vi "Emballage_fichierSpecifique_S0020002_HTML.vi"(5 "Indice Rev. Client":string, 6 "Logo IMI (U:\\MTD_PRD_TESTS\\PARAM_TESTS\\EMBALLAGE\\LogoIMI.JPG)":path=path "U:/MTD_PRD_TESTS/PARAM_TESTS/EMBALLAGE/LogoIMI.JPG", 7 "N° article client":string, 8 "Error in":errorcluster caption="Error in (no error)", 9 "PDF filename path":path=path "C:/Users/ltinguely/Desktop/test.pdf", 10 "report file path":path=path "C:/Users/ltinguely/Desktop/test.html" caption="chemin du fichier du rapport", 11 "Tableau n° valves":string[](array[string])=["100200021121130326", "100200021121130308", "100200021121130314", "100200021121130316", "100200021121130319", "100200021121130330", "100200021121130309", "100200021121130307", "100200021121130311", "100200021121130299", "100200021121130310", "100200021121130313", "100200021121130321", "100200021121130336", "100200021121130322", "100200021121130302", "100200021121130334", "100200021121130317", "100200021121130348", "100200021121130333", "100200021121130355", "100200021121130345", "100200021121130349", "100200021121130350", "100200021121130315", "100200021121130352", "100200021121130328", "100200021121130337", "100200021121130357", "100200021121130359", "100200021121130360", "100200021121130344", "100200021121130347", "100200021121130358", "100200021121130341", "100200021121130338", "100200021121130331", "100200021121130329", "100200021121130332", "100200021121130339", "100200021121130340", "100200021121130343", "100200021121130351", "100200021121130354", "100200021121130346", "100200021121130335", "100200021121130342", "100200021121130353", "100200021121130383", "100200021121130384", "100200021121130380", "100200021121130389", "100200021121130382", "100200021121130379", "100200021121130376", "100200021121130378", "100200021121130391", "100200021121130392", "100200021121130372", "100200021121130362", "100200021121130375", "100200021121130371", "100200021121130385", "100200021121130364", "100200021121130386", "100200021121130361", "100200021121130366", "100200021121130365", "100200021121130367", "100200021121130363", "100200021121130377", "100200021121130374", "100200021121130369", "100200021121130370", "100200021121130373", "100200021121130388", "100200021121130368", "100200021121130356", "100200021121130412", "100200021121130407", "100200021121130406", "100200021121130408", "100200021121130398", "100200021121130415", "100200021121130402", "100200021121130399", "100200021121130414", "100200021121130413", "100200021121130393", "100200021121130390", "100200021121130403", "100200021121130401", "100200021121130387", "100200021121130381", "100200021121130395", "100200021121130394", "100200021121130411", "100200021121130410", "100200021121130405", "100200021121130396", "100200021121130397", "100200021121130400", "100200021121130404", "100200021121130211", "100200021121130215", "100200021121130217", "100200021121130212", "100200021121130219", "100200021121130225", "100200021121130213", "100200021121130216", "100200021121130226", "100200021121130224", "100200021121130223", "100200021121130230", "100200021121130220", "100200021121130214", "100200021121130229", "100200021121130236", "100200021121130238", "100200021121130239", "100200021121130237", "100200021121130234", "100200021121130242", "100200021121130241", "100200021121130233", "100200021121130210", "100200021121130218", "100200021121130240", "100200021121130221", "100200021121130245", "100200021121130222", "100200021121130235", "100200021121130247", "100200021121130227", "100200021121130231", "100200021121130228", "100200021121130243", "100200021121130246", "100200021121130251", "100200021121130273", "100200021121130267", "100200021121130268", "100200021121130256", "100200021121130265", "100200021121130261", "100200021121130264", "100200021121130254", "100200021121130257", "100200021121130249", "100200021121130248", "100200021121130250", "100200021121130244", "100200021121130253", "100200021121130266", "100200021121130252", "100200021121130274", "100200021121130263", "100200021121130232", "100200021121130262", "100200021121130260", "100200021121130269", "100200021121130270", "100200021121130294", "100200021121130255", "100200021121130258", "100200021121130295", "100200021121130297", "100200021121130291", "100200021121130289", "100200021121130278", "100200021121130283", "100200021121130284", "100200021121130296", "100200021121130277", "100200021121130286", "100200021121130288", "100200021121130287", "100200021121130275", "100200021121130290", "100200021121130298", "100200021121130279", "100200021121130292", "100200021121130259", "100200021121130293", "100200021121130272", "100200021121130271", "100200021121130276", "100200021121130282", "100200021121130281", "100200021121130280", "100200021121130285", "100200021121130300", "100200021121130152", "100200021121130165", "100200021121130178", "100200021121130151", "100200021121130175", "100200021121130173", "100200021121130157", "100200021121130167", "100200021121130155", "100200021121130174", "100200021121130164", "100200021121130163", "100200021121130159", "100200021121130160", "100200021121130186", "100200021121130154", "100200021121130169", "100200021121130166", "100200021121130156", "100200021121130207", "100200021121130192", "100200021121130158", "100200021121130161", "100200021121130168", "100200021121130170", "100200021121130171", "100200021121130162", "100200021121130190", "100200021121130191", "100200021121130193", "100200021121130182", "100200021121130183", "100200021121130176", "100200021121130148", "100200021121130177", "100200021121130203", "100200021121130184", "100200021121130189", "100200021121130194", "100200021121130179", "100200021121130196", "100200021121130188", "100200021121130180", "100200021121130187", "100200021121130181", "100200021121130195", "100200021121130185", "100200021121130204", "100200021121130202", "100200021121130200", "100200021121130198", "100200021121130197", "100200021121130199", "100200021121130150", "100200021121130111", "100200021121130201", "100200021121130208", "100200021121130209", "100200021121130205", "100200021121130206", "100200021121130093", "100200021121130091", "100200021121130109", "100200021121130088", "100200021121130099", "100200021121130097", "100200021121130096", "100200021121130102", "100200021121130095", "100200021121130092", "100200021121130094", "100200021121130098", "100200021121130101", "100200021121130100", "100200021121130106", "100200021121130121", "100200021121130104", "100200021121130107", "100200021121130089", "100200021121130103", "100200021121130105", "100200021121130108", "100200021121130120", "100200021121130125", "100200021121130138", "100200021121130114", "100200021121130115", "100200021121130119", "100200021121130118", "100200021121130117", "100200021121130113", "100200021121130112", "100200021121130124", "100200021121130110", "100200021121130116", "100200021121130149", "100200021121130145", "100200021121130127", "100200021121130130", "100200021121130128", "100200021121130129", "100200021121130134", "100200021121130133", "100200021121130135", "100200021121130143", "100200021121130139", "100200021121130147", "100200021121130136", "100200021121130141", "100200021121130144", "100200021121130126", "100200021121130123", "100200021121130122", "100200021121130132", "100200021121130131", "100200021121130140", "100200021121130146", "100200021121130137", "100200021121130142", "100200021121130153", "100200021121130060", "100200021121130077", "100200021121130059", "100200021121130040", "100200021121130075", "100200021121130082", "100200021121130022", "100200021121130086", "100200021121130045", "100200021121130078", "100200021121130080", "100200021121130074", "100200021121130065", "100200021121130066", "100200021121130070", "100200021121130068", "100200021121130084", "100200021121130069", "100200021121130076", "100200021121130081", "100200021121130083", "100200021121130085", "100200021121130087", "100200021121130090", "100200021121130012", "100200021121130028", "100200021121130079", "100200021121130073", "100200021121130072", "100200021121130071", "100200021121130042", "100200021121130030", "100200021121130033", "100200021121130032", "100200021121130027", "100200021121130031", "100200021121130025", "100200021121130020", "100200021121130026", "100200021121130003", "100200021121130008", "100200021121130001", "100200021121130019", "100200021121120509", "100200021121130021", "100200021121130016", "100200021121130013", "100200021121120510", "100200021121130015", "100200021121130002", "100200021121130014", "100200021121130029", "100200021121130049", "100200021121130048", "100200021121130011", "100200021121130063", "100200021121130009", "100200021121130010", "100200021121130004", "100200021121130017", "100200021121130018", "100200021121130024", "100200021121130023", "100200021121130061", "100200021121130062", "100200021121130064", "100200021121130058", "100200021121130046", "100200021121130056", "100200021121130057", "100200021121130054", "100200021121130051", "100200021121130044", "100200021121130035", "100200021121130043", "100200021121130005", "100200021121130038", "100200021121130039", "100200021121130047", "100200021121130053", "100200021121130007", "100200021121130037", "100200021121130006", "100200021121130052", "100200021121130041", "100200021121130034", "100200021121130036", "100200021121130067", "100200021121130050", "100200021121130055", "100200021121120410", "100200021121120406", "100200021121120421", "100200021121120408", "100200021121120424", "100200021121120416", "100200021121120423", "100200021121120419", "100200021121120407", "100200021121120397", "100200021121120396", "100200021121120404", "100200021121120422", "100200021121120392", "100200021121120403", "100200021121120405", "100200021121120400", "100200021121120385", "100200021121120348", "100200021121120388", "100200021121120414", "100200021121120412", "100200021121120320", "100200021121120394", "100200021121120447", "100200021121120398", "100200021121120444", "100200021121120417", "100200021121120395", "100200021121120402", "100200021121120401", "100200021121120393", "100200021121120399", "100200021121120425", "100200021121120449", "100200021121120415", "100200021121120446", "100200021121120439", "100200021121120426", "100200021121120434", "100200021121120453", "100200021121120455", "100200021121120441", "100200021121120443", "100200021121120435", "100200021121120409", "100200021121120420", "100200021121120427", "100200021121120429", "100200021121120438", "100200021121120432", "100200021121120437", "100200021121120430", "100200021121120440", "100200021121120442", "100200021121120428", "100200021121120464", "100200021121120433", "100200021121120418", "100200021121120445", "100200021121120431", "100200021121120463", "100200021121120451", "100200021121120466", "100200021121120454", "100200021121120452", "100200021121120459", "100200021121120411", "100200021121120458", "100200021121120472", "100200021121120470", "100200021121120474", "100200021121120462", "100200021121120477", "100200021121120436", "100200021121120469", "100200021121120467", "100200021121120413", "100200021121120460", "100200021121120486", "100200021121120476", "100200021121120473", "100200021121120468", "100200021121120478", "100200021121120482", "100200021121120471", "100200021121120479", "100200021121120456", "100200021121120465", "100200021121120461", "100200021121120488", "100200021121120457", "100200021121120475", "100200021121120489", "100200021121120493", "100200021121120487", "100200021121120485"]) -> (0 "Error out":errorcluster, 1 "report out":refnum<class "NI_report.lvclass"> caption="rapport en sortie", 2 "path out":path, 3 "IsSuccessful":bool)   [LabVIEW 2020]
uses:
  <vilib>/Utility/NIReport.llb/NI_report.lvclass
  <vilib>/Utility/NIReport.llb/Report Type.ctl
  <vilib>/printing/OpenHTMLReport.llb/Open HTML Report in Browser (Refnum).vi
  <vilib>/Utility/NIReport.llb/NI_ReportGenerationCore.lvlib
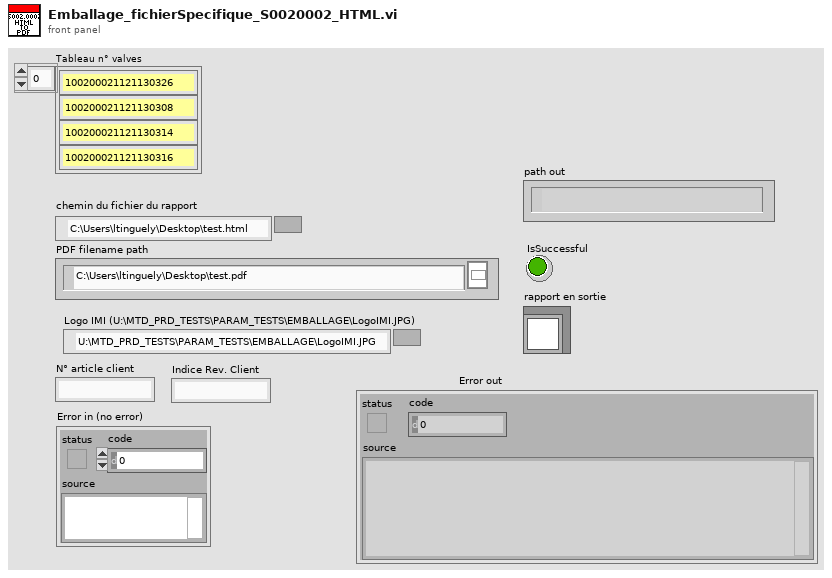
[diagram p1: front panel]
types:
  T1 = typedef "NI_ReportGenerationCore.lvlib/Report Type.ctl" = enum16{"HTML", "Word", "Excel"}
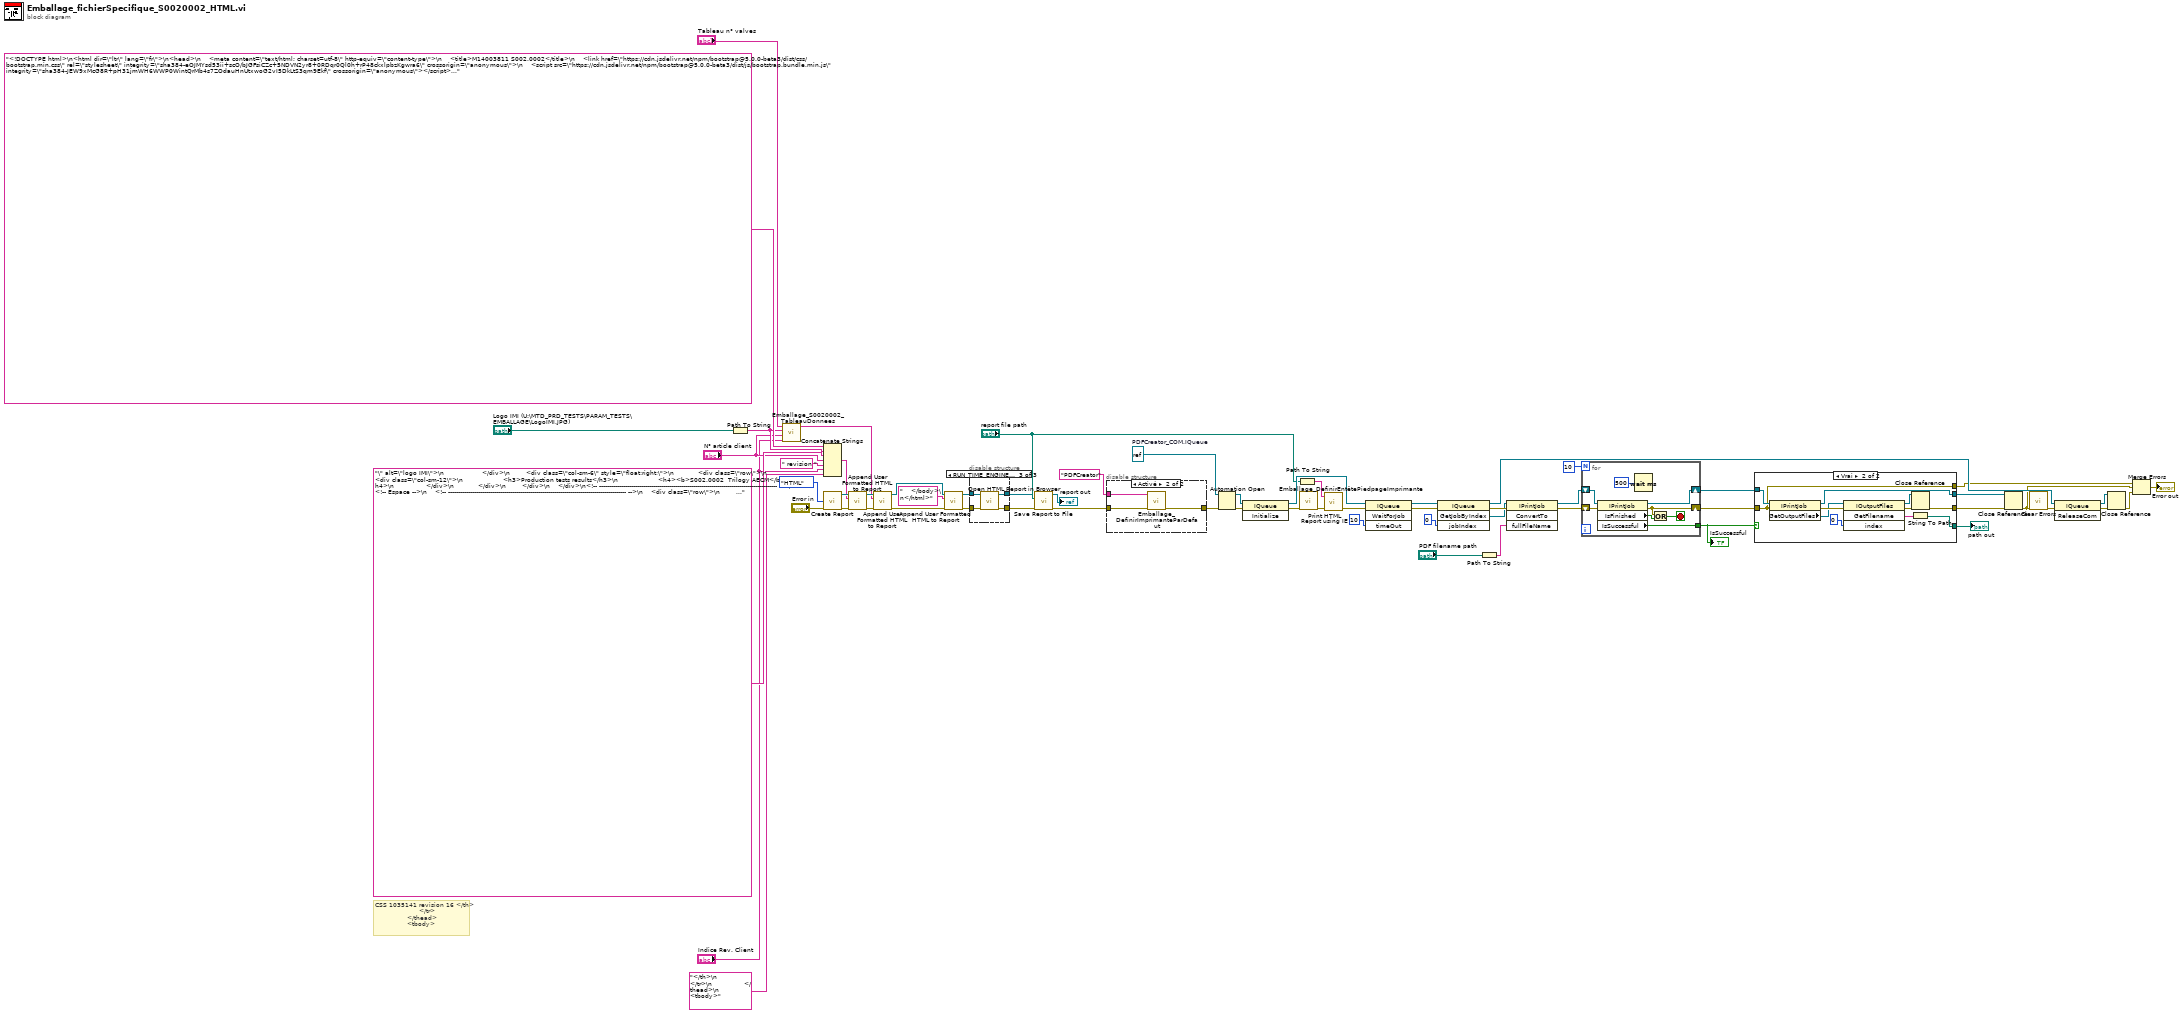
[diagram p0: block diagram]
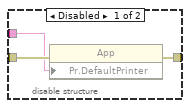
[diagram p2: hidden frame]
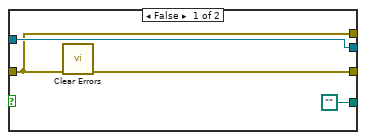
[diagram p5: hidden frame]
diagram:
  w52 = refnum<k7> refnum  # PDFCreator_COM.IQueue
  # "CSS 1035141 revision 16 </th>\n                      </tr>\n                </thead>\n                <tbody>"
  n1 = Path To String(path="Logo IMI (U:\\MTD_PRD_TESTS\\PARAM_TESTS\\EMBALLAGE\\LogoIMI.JPG)") -> (string=w20:string)
  n2 = call "Emballage_S0020002_TableauDonnees.vi"("Indice Rev Client"="Indice Rev. Client", "N° article client"="N° article client", "Chemin Logo"=w20, "Tableau n° valves"="Tableau n° valves") -> ("Chaîne en sortie"=w28:string)  [unwired: 7 in]
  n3 = Concatenate Strings("<!DOCTYPE html>\n<html dir=\"ltr\" lang=\"fr\">\n<head>\n    <meta content=\"text/html; charset=utf-8\" http-equiv=\"content-type\">\n    <title>M14003811 S002.0002</title>\n    <link href=\"https://cdn.jsdelivr.net/npm/bootstrap@5.0.0-beta3/dist/css/bootstrap.min.css\" rel=\"stylesheet\" integrity=\"sha384-eOJMYsd53ii+scO/bJGFsiCZc+5NDVN2yr8+0RDqr0Ql0h+rP48ckxlpbzKgwra6\" crossorigin=\"anonymous\">\n    <script src=\"https://cdn.jsdelivr.net/npm/bootstrap@5.0.0-beta3/dist/js/bootstrap.bundle.min.js\" integrity=\"sha384-JEW9xMcG8R+pH31jmWH6WWP0WintQrMb4s7ZOdauHnUtxwoG2vI5DkLtS3qm9Ekf\" crossorigin=\"anonymous\"></script>\n<style>\n        @media all {\n    table {\n        margin: auto;\n    }\n    table,\n    th,\n    td {\n        padding: 1px;\n        border: 1px solid black;\n        border-collapse: collapse;\ntext-align: center;\n    }\n}\n@media print {\ntable{\ndisplay:table !important;\n    width:80%;\n    margin-left:10%;\n}\n}\n      </style>\n       <meta content=\"LTinguely\" name=\"author\">\n    <meta content=\"M14003811\" name=\"description\">\n    <meta content=\"M14003811\" name=\"keywords\">\n</head>\n<body>\n    <!-- ----------------------------------------------------------------------------------------- -->\n    <!-- Titre -->\n    <!-- ----------------------------------------------------------------------------------------- -->\n     <div class=\"row\" style=\"display: inline-block\">\n        <div class=\"col-sm-6\" style=\"float:left;\">\n                            <img src=\"", w20, "\" alt=\"logo IMI\">\n                   </div>\n        <div class=\"col-sm-6\" style=\"float:right;\">\n            <div class=\"row\">\n                <div class=\"col-sm-12\">\n                    <h3>Production tests results</h3>\n                    <h4><b>S002.0002  Trilogy AECM</b></h4>\n                </div>\n            </div>\n        </div>\n    </div>\n<!-- ----------------------------------------------------------------------------------------- -->\n    <!-- Espace -->\n    <!-- ----------------------------------------------------------------------------------------- -->\n    <div class=\"row\">\n        <div class=\"col-sm-12\">\n            <br>\n            <br>\n        </div>\n    </div>\n    <!-- ----------------------------------------------------------------------------------------- -->\n    <!-- Explciation Fichier Encadrée -->\n    <!-- ----------------------------------------------------------------------------------------- -->\n    <div class=\"row border border-dark\">\n        <div class=\"col-sm-12\">\n            <p style=\"font-weight: bold;\">This document is a complementory document to the Certificate of Conformity.<br>\n            This document states the test result status (Pass or Fail) for each parts serial number for which\n            the associated certificate of Conformity was issued</p>\n        </div>\n    </div>\n    <!-- ----------------------------------------------------------------------------------------- -->\n    <!-- Espace -->\n    <!-- ----------------------------------------------------------------------------------------- -->\n    <div class=\"row\">\n        <div class=\"col-sm-12\">\n            <br>\n            <br>\n        </div>\n    </div>\n    <!-- ----------------------------------------------------------------------------------------- -->\n    <!-- Données -->\n    <!-- ----------------------------------------------------------------------------------------- -->\n    \n            <table>\n                <thead>\n                    <tr>\n                        <th></th>\n                        <th>Serial Number</th>\n                        <th>Test results according to<br>" ("HTML text"), "N° article client", " revision " ("chaîne"), "Indice Rev. Client", "</th>\n                      </tr>\n                </thead>\n                <tbody>" ("chaîne")) -> (w24:string)
  n4 = call <vilib>:"Create Report.vi"("report type"=Report_Type."HTML", "error in (no error)"="Error in") -> ("report out"=w25:refnum<class "NI_report.lvclass">, "error out"=w26:errorcluster)  [unwired: 12 in]
  n5 = call-dynamic "Append User Formatted HTML to Report.vi"("report in"=w25, "HTML text"=w24, "error in (no error)"=w26) -> ("report out"=w59:refnum<class "NI_report.lvclass">, "error out"=w60:errorcluster)  [unwired: 11 in]
  n6 = call-dynamic "Append User Formatted HTML to Report.vi"("report in"=w59, "HTML text"=w28, "error in (no error)"=w60) -> ("report out"=w58:refnum<class "NI_report.lvclass">, "error out"=w57:errorcluster)  [unwired: 11 in]
  n7 = call-dynamic "Append User Formatted HTML to Report.vi"("report in"=w58, "HTML text"="    </body>\n</html>", "error in (no error)"=w57) -> ("report out"=w19:refnum<class "NI_report.lvclass">, "error out"=w18:errorcluster)  [unwired: 11 in]
  n8 = disable-structure shown="RUN_TIME_ENGINE==False" {
    disable-tunnel: w19 -> [w64 w66 w70]
    disable-tunnel: w18 -> [w63 w65 w69]
    disable-tunnel: [w64 w66 w68] -> w17
    disable-tunnel: [w63 w65 w67] -> w16
    frame condition #0 {
    }
    frame condition #1 {
    }
    frame condition #2 (active) {
      n9 = call-poly <vilib>:"Open HTML Report in Browser.vi"("report in"=w70, "error in (no error)"=w69) -> ("report out"=w68:refnum<class "NI_report.lvclass">, "error out"=w67:errorcluster)  [unwired: 11 in, 1 out]
    }
  }
  n10 = call-dynamic "Save Report to File.vi"("report in"=w17, "report file path"="report file path", "error in (no error)"=w16) -> ("report out"=→"report out":refnum<class "NI_report.lvclass">, "error out"=w6:errorcluster)  [unwired: 11 in]
  n11 = disable-structure shown="Activé" {
    disable-tunnel: [w73 w74] -> w53
    disable-tunnel: w6 -> [w72 w75]
    disable-tunnel: "PDFCreator" ("Printing:Default Printer") -> [w71 w76]
    frame Disabled {
      n12 = property class="App"(error in=w72, "Pr.DefaultPrinter"=w71) -> (error out=w73:errorcluster)  [unwired: 1 in, 1 out]
    }
    frame Enabled {
      n13 = call "Emballage_DefinirImprimanteParDefaut.vi"("Error in"=w75, "Imprimante"=w76) -> ("Error out"=w74:errorcluster)  [unwired: 9 in]
    }
  }
  n14 = Automation Open(error in (no error)=w53, Automation Refnum=w52) -> (Automation Refnum=w14:refnum<k7>, error out=w46:errorcluster)  [unwired: 2 in]
  n15 = invoke class="IQueue" method="Initialize"(reference=w14, error in=w46) -> (reference out=w47:refnum<k7>, error out=w8:errorcluster)  [unwired: 1 in, 1 out]
  n16 = Path To String(path="report file path") -> (string=w27:string)
  n17 = call "Emballage_DefinirEntêtePiedpageImprimante.vi"("Error in"=w8) -> ("Error out"=w7:errorcluster)  [unwired: 10 in]
  n18 = call <vilib>:"Print HTML Report using IE.vi"("error in (no error)"=w7, "path to HTML"=w27) -> ("error out"=w33:errorcluster)  [unwired: 3 out]
  n19 = invoke class="IQueue" method="WaitForJob"(reference=w47, error in=w33, "timeOut"=10 ("Time out (sec)")) -> (reference out=w11:refnum<k7>, error out=w13:errorcluster)  [unwired: 1 in, 2 out]
  n20 = invoke class="IQueue" method="GetJobByIndex"(reference=w11, error in=w13, "jobIndex"=0 ("jobIndex (0)")) -> (reference out=w45:refnum<k7>, error out=w49:errorcluster, "GetJobByIndex"=w15:refnum<k7>)  [unwired: 1 in, 1 out]
  n21 = Path To String(path="PDF filename path") -> (string=w54:string)
  n22 = invoke class="IPrintJob" method="ConvertTo"(reference=w15, error in=w49, "fullFileName"=w54) -> (reference out=w43:refnum<k7>, error out=w41:errorcluster)  [unwired: 1 in, 2 out]
  n23 = for {
    N: 10 -> [_]
    shift-right: [w83] -> w42
    shift-left: w43 -> [w84]
    shift-right: [w79] -> w39
    shift-left: w41 -> [w82]
    tunnel: [w81] -> w37
    stop <- w77 stop-if-true
    n24 = property class="IPrintJob"(reference=w84, error in=w82) -> (reference out=w83:refnum<k7>, error out=w79:errorcluster, "IsFinished"=w78:bool, "IsSuccessful"=w81:bool)
    n25 = Wait (ms)(milliseconds to wait=u32 500) -> ()  [unwired: 1 out]
    n26 = Or(x=w79, y=w78) -> (x .or. y?=w77:bool)
  }
  "IsSuccessful" <- w37
  n27 = case shown="Vrai" w37 {
    tunnel: [w88 w99] -> w44
    tunnel: w42 -> [w88 w98]
    tunnel: w39 -> [w85 w89]
    tunnel: [w86 w93] -> w38
    tunnel: [path "" w91] -> w35
    tunnel: [w85 w89] -> w29
    frame False {
      n28 = call <vilib>:"Clear Errors.vi"("error in (no error)"=w85) -> ("error out"=w86:errorcluster)  [unwired: 5 in, 1 out]
    }
    frame True {
      n29 = property class="IPrintJob"(reference=w98, error in=w89) -> (reference out=w99:refnum<k7>, error out=w96:errorcluster, "GetOutputFiles"=w90:refnum<k7>)
      n30 = invoke class="IOutputFiles" method="GetFilename"(reference=w90, error in=w96, "index"=0) -> (reference out=w94:refnum<k7>, error out=w95:errorcluster, "GetFilename"=w92:string)  [unwired: 1 in, 1 out]
      n31 = String To Path(string=w92) -> (path=w91:path)
      n32 = Close Reference(reference=w94, error in (no error)=w95) -> (error out=w93:errorcluster)
    }
  }
  "path out" <- w35
  n33 = Close Reference(reference=w44, error in (no error)=w38) -> (error out=w30:errorcluster)
  n34 = call <vilib>:"Clear Errors.vi"("error in (no error)"=w30) -> ("error out"=w31:errorcluster)  [unwired: 5 in, 1 out]
  n35 = invoke class="IQueue" method="ReleaseCom"(reference=w45, error in=w31) -> (reference out=w50:refnum<k7>, error out=w51:errorcluster)  [unwired: 1 in, 1 out]
  n36 = Close Reference(reference=w50, error in (no error)=w51) -> (error out=w34:errorcluster)
  n37 = Merge Errors(w29, w30, w34) -> (→"Error out":errorcluster)
